vi "VI Tree.vi"   [LabVIEW 2010, in "Stanford Research 844.lvlib"]
doc: "This is the instrument driver for the Stanford Research Systems SR844, Lock-In Amplifier. The VI Tree displays all the user-callable VIs of the instrument driver in an organized table."
uses:
  <instrlib>/Stanford Research 844/Stanford Research 844.lvlib
panel:
  # "© 2005 National Instruments.  ALL RIGHTS RESERVED."
  # "SEE DIAGRAM\nFOR VI TREE."
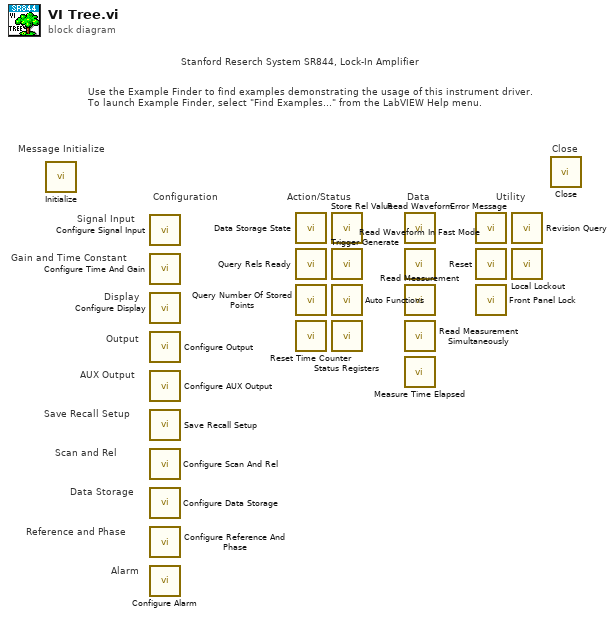
[diagram p0: block diagram]
diagram:
  # "Display"
  # "Alarm"
  # "Scan and Rel"
  # "Data Storage"
  # "Save Recall Setup"
  # "AUX Output"
  # "Output"
  # "Gain and Time Constant"
  # "Signal Input"
  # "Reference and Phase"
  # "Stanford Reserch System SR844, Lock-In Amplifier"
  # "Use the Example Finder to find examples demonstrating the usage of this instrument driver.\nTo launch Example Finder, select \"Find Examples...\" from the LabVIEW Help menu."
  # "Configuration"
  # "Utility"
  # "Data"
  # "Action/Status"
  # "Close"
  # "Message Initialize"
  n1 = call <instrlib>:"Initialize.vi"() -> ()  [unwired: 10 in, 2 out]
  n2 = call <instrlib>:"Configure Signal Input.vi"() -> ()  [unwired: 10 in, 2 out]
  n3 = call <instrlib>:"Configure Time And Gain.vi"() -> ()  [unwired: 14 in, 2 out]
  n4 = call <instrlib>:"Configure Display.vi"() -> ()  [unwired: 10 in, 2 out]
  n5 = call <instrlib>:"Configure Output.vi"() -> ()  [unwired: 18 in, 2 out]
  n6 = call <instrlib>:"Configure AUX Output.vi"() -> ()  [unwired: 10 in, 2 out]
  n7 = call <instrlib>:"Save Recall Setup.vi"() -> ()  [unwired: 10 in, 2 out]
  n8 = call <instrlib>:"Configure Scan And Rel.vi"() -> ()  [unwired: 10 in, 2 out]
  n9 = call <instrlib>:"Configure Data Storage.vi"() -> ()  [unwired: 10 in, 2 out]
  n10 = call <instrlib>:"Configure Reference And Phase.vi"() -> ()  [unwired: 10 in, 2 out]
  n11 = call <instrlib>:"Configure Alarm.vi"() -> ()  [unwired: 10 in, 2 out]
  n12 = call <instrlib>:"Data Storage State.vi"() -> ()  [unwired: 10 in, 2 out]
  n13 = call <instrlib>:"Query Rels Ready.vi"() -> ()  [unwired: 9 in, 3 out]
  n14 = call <instrlib>:"Query Number Of Stored Points.vi"() -> ()  [unwired: 9 in, 3 out]
  n15 = call <instrlib>:"Reset Time Counter.vi"() -> ()  [unwired: 10 in, 2 out]
  n16 = call <instrlib>:"Store Rel Value.vi"() -> ()  [unwired: 10 in, 2 out]
  n17 = call <instrlib>:"Trigger Generate.vi"() -> ()  [unwired: 10 in, 2 out]
  n18 = call <instrlib>:"Auto Functions.vi"() -> ()  [unwired: 18 in, 2 out]
  n19 = call <instrlib>:"Status Registers.vi"() -> ()  [unwired: 9 in, 3 out]
  n20 = call <instrlib>:"Read Waveform.vi"() -> ()  [unwired: 9 in, 3 out]
  n21 = call <instrlib>:"Read Waveform In Fast Mode.vi"() -> ()  [unwired: 8 in, 4 out]
  n22 = call <instrlib>:"Read Measurement.vi"() -> ()  [unwired: 9 in, 3 out]
  n23 = call <instrlib>:"Read Measurement Simultaneously.vi"() -> ()  [unwired: 9 in, 3 out]
  n24 = call <instrlib>:"Measure Time Elapsed.vi"() -> ()  [unwired: 9 in, 3 out]
  n25 = call <instrlib>:"Error Message.vi"() -> ()  [unwired: 11 in, 5 out]
  n26 = call <instrlib>:"Reset.vi"() -> ()  [unwired: 14 in, 2 out]
  n27 = call <instrlib>:"Front Panel Lock.vi"() -> ()  [unwired: 10 in, 2 out]
  n28 = call <instrlib>:"Revision Query.vi"() -> ()  [unwired: 12 in, 4 out]
  n29 = call <instrlib>:"Local Lockout.vi"() -> ()  [unwired: 10 in, 2 out]
  n30 = call <instrlib>:"Close.vi"() -> ()  [unwired: 11 in, 1 out]
